vi "Point2Rect.vi"(8 "错误输入":errorcluster, 10 "point b":cluster{"x":dbl, "y":dbl} caption="点b" {"y" format="%.2f"; "x" format="%.2f"}, 11 "point a":cluster{"x":dbl, "y":dbl} caption="点a" {"y" format="%.2f"; "x" format="%.2f"}) -> (0 "错误输出":errorcluster, 3 "rect":T1 caption="矩形")   [LabVIEW 2012, in "Rect Tools.lvlib"]
uses:
  Rect Tools.lvlib
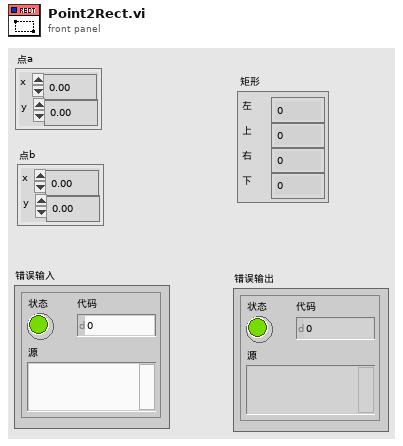
[diagram p1: front panel]
types:
  T1 = cluster{"left":i16, "top":i16, "right":i16, "bottom":i16}
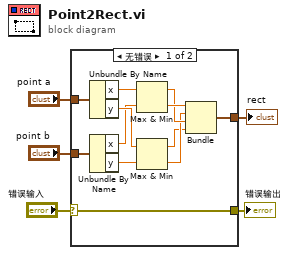
[diagram p0: block diagram]
diagram:
  n1 = case shown="无错误" "错误输入" {
    selector: "错误输入" -> [w9 w18]
    tunnel: [w9 w18] -> w4
    tunnel: "point a" -> [w8 _]
    tunnel: "point b" -> [w7 _]
    tunnel: [w6 _] -> w1
    frame No Error {
      n2 = Unbundle By Name(w8) -> ("x"=w17:dbl, "y"=w14:dbl)
      n3 = Unbundle By Name(w7) -> ("x"=w10:dbl, "y"=w13:dbl)
      n4 = Max & Min(x=w17, y=w10) -> (max(x,y)=w15:dbl, min(x,y)=w16:dbl)
      n5 = Max & Min(x=w14, y=w13) -> (max(x,y)=w11:dbl, min(x,y)=w12:dbl)
      n6 = Bundle(w16, w12, w15, w11) -> (w6:cluster{dbl, dbl, dbl, dbl})  [unwired: 1 in]
    }
    frame Error {
    }
  }
  "错误输出" <- w4
  "rect" <- w1
